vi "Example.vi"() -> ()   [LabVIEW 2014]
uses:
  PPT.lvclass
  reusable/Session APIs/File Access/Config Data/Config Data.lvclass
  reusable/Session APIs/File Access/Config Data/Config Data.lvclass/Config Data.ctl
  Configurable Device/Configurable Device.lvclass/Configurable Device.ctl
  PPT.lvclass/PPT.ctl
  reusable/Data/Array Data/2D Single/2D Single Data.lvclass
  reusable/Session APIs/File Access/Config Data/Accessors/Write Cfg Path.vi
  Configurable Device/Write Handle.vi
  Accessors/Write IDs.vi
  <userlib>/_Session Fwk/Session - Root.lvclass
panel:
  out "error out 2":errorcluster
  out "Data":sgl[][](array[numeric])
  out "error out":errorcluster
  in  "milliseconds to wait":u32
  in  "Stop Button":bool
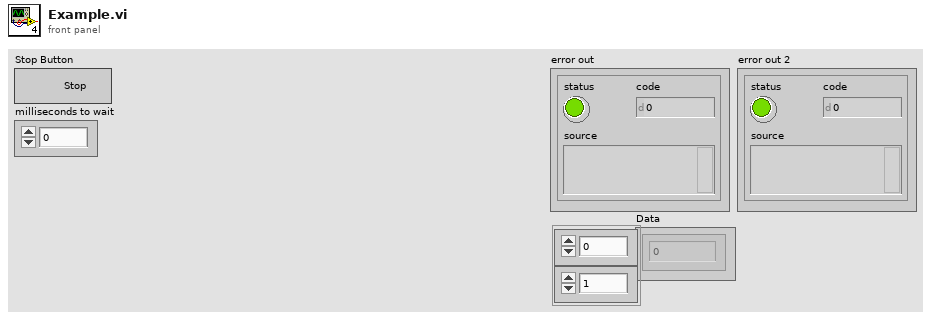
[diagram p1: front panel]
types:
  T1 = typedef "Session - Root.lvclass/Session Handle.ctl" = refnum<data-value>
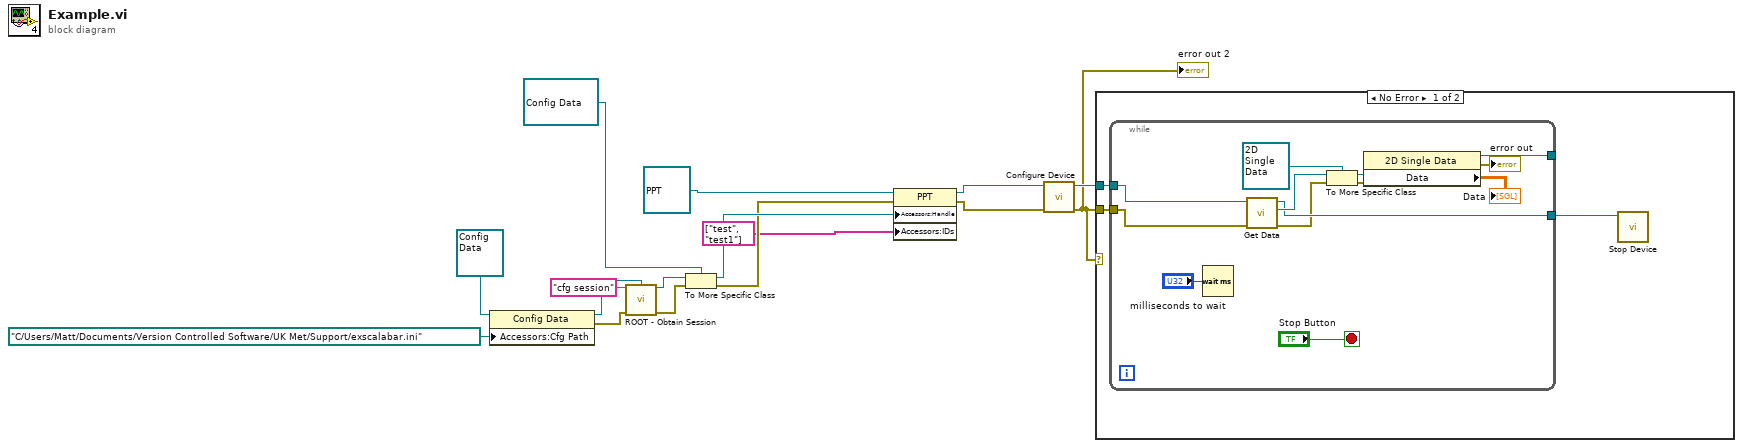
[diagram p0: block diagram]
diagram:
  n1 = property class="Config Data"(reference=refnum<class "Config Data.lvclass"> refnum ("Config Data"), "Accessors:Cfg Path"=path "C:/Users/Matt/Documents/Version Controlled Software/UK Met/Support/exscalabar.ini" ("Cfg Path")) -> (reference out=w13:refnum<class "Config Data.lvclass">, error out=w3:errorcluster)  [unwired: 1 in]
  n2 = call <userlib>:"ROOT - Obtain Session.vi"("Session Name ()"="cfg session", "OBJ - Session"=w13, "error in (no error)"=w3) -> ("Session Handle"=w11:T1, "error out"=w2:errorcluster)  [unwired: 10 in, 1 out]
  n3 = To More Specific Class(target class=refnum<data-value> refnum ("Session Handle"), reference=w11, error in=w2) -> (specific class reference=w9:refnum<data-value>, error out=w8:errorcluster)
  n4 = property class="PPT"(reference=refnum<class "PPT.lvclass"> refnum ("PPT"), error in=w8, "Accessors:Handle"=w9, "Accessors:IDs"=string[] ["test", "test1"] ("IDs")) -> (reference out=w6:refnum<class "PPT.lvclass">, error out=w5:errorcluster)
  n5 = call-dynamic "Configure Device.vi"("error in"=w5, "PPT in"=w6) -> ("error out"=w1:errorcluster, "PPT out"=w4:refnum<class "PPT.lvclass">)  [unwired: 8 in]
  "error out 2" <- w1
  n6 = case shown="No Error" w1 {
    tunnel: w4 -> [w19 _]
    tunnel: w1 -> [w18 _]
    frame No Error {
      n7 = while {
        tunnel: w19 -> [w30]
        tunnel: w18 -> [w29]
        tunnel: [w25] -> _
        tunnel: [w24] -> w17
        stop <- "Stop Button" stop-if-true
        n8 = Wait (ms)(milliseconds to wait="milliseconds to wait") -> ()  [unwired: 1 out]
        n9 = call-dynamic "Get Data.vi"("error in"=w29, "PPT in"=w30) -> ("error out"=w23:errorcluster, "DataOut"=w28:refnum<class "Data.lvclass">, "PPT out"=w24:refnum<class "PPT.lvclass">)  [unwired: 7 in]
        n10 = To More Specific Class(target class=refnum<class "2D Single Data.lvclass"> refnum ("Base Data Lib:2D Single Data"), reference=w28, error in=w23) -> (specific class reference=w26:refnum<class "2D Single Data.lvclass">, error out=w22:errorcluster)
        n11 = property class="2D Single Data"(reference=w26, error in=w22) -> (reference out=w25:refnum<class "2D Single Data.lvclass">, error out=→"error out":errorcluster, "Data"=→"Data":sgl[][])
      }
      n12 = call-dynamic "Stop Device.vi"("PPT in"=w17) -> ()  [unwired: 9 in, 2 out]
    }
    frame Error {
    }
  }
